vi "read_params.vi"(8 "error in (no error)":errorcluster, 11 "OrthogonalMatchingPursuitCV in":refnum<class "OrthogonalMatchingPursuitCV.lvclass">) -> (0 "error out":errorcluster, 2 "params":T1={"copy"=TRUE, "fit_intercept"=TRUE, "normalize"=TRUE, "max_iter"={"max_iter_type"="None", "max_iter_int"=0.0}, "cv"=5.0, "n_jobs"=1.0, "verbose"={"verbose_type"="bool", "verbose_bool"=FALSE, "verbose_int"=0.0}}, 3 "OrthogonalMatchingPursuitCV out":refnum<class "OrthogonalMatchingPursuitCV.lvclass">)   [LabVIEW 2020, in "OrthogonalMatchingPursuitCV.lvclass"]
uses:
  OrthogonalMatchingPursuitCV.lvclass
  Controls/orthogonal_matching_pursuit_cv_params.ctl
  OrthogonalMatchingPursuitCV.lvclass/OrthogonalMatchingPursuitCV.ctl
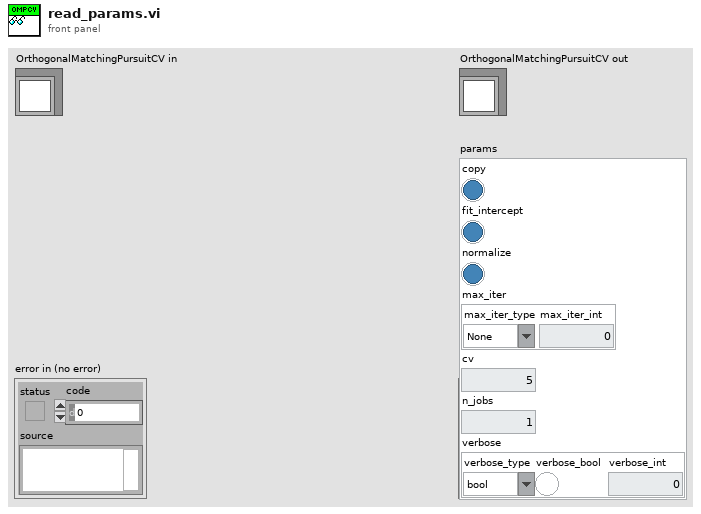
[diagram p1: front panel]
types:
  T1 = typedef "orthogonal_matching_pursuit_cv_params.ctl" = cluster{"copy":bool, "fit_intercept":bool, "normalize":bool, "max_iter":cluster{"max_iter_type":string, "max_iter_int":dbl}, "cv":dbl, "n_jobs":dbl, "verbose":cluster{"verbose_type":string, "verbose_bool":bool, "verbose_int":dbl}}
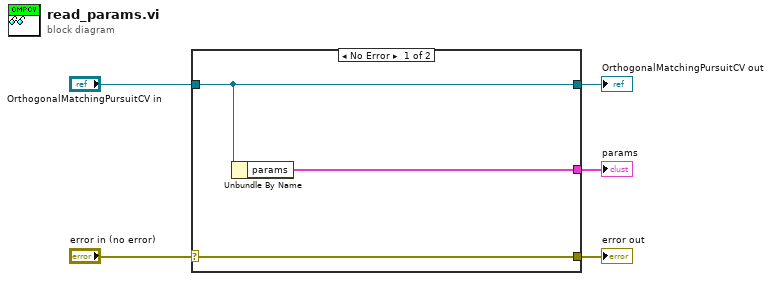
[diagram p0: block diagram]
diagram:
  n1 = case shown="No Error" "error in (no error)" {
    selector: "error in (no error)" -> [w8 w9]
    tunnel: [w8 w9] -> w4
    tunnel: [w7 w10] -> w2
    tunnel: "OrthogonalMatchingPursuitCV in" -> [w7 w10]
    tunnel: [w6 _] -> w1
    frame No Error {
      n2 = Unbundle By Name(w7) -> ("params"=w6:T1)
    }
    frame Error {
    }
  }
  "error out" <- w4
  "OrthogonalMatchingPursuitCV out" <- w2
  "params" <- w1
